vi "test Add State.vi"(8 "error in (no error)":errorcluster, 11 "TestCase in":refnum<class "Switch Scripting Unit Tests.lvclass">) -> (0 "error out":errorcluster, 3 "TestCase out":refnum<class "Switch Scripting Unit Tests.lvclass">)   [LabVIEW 2017, in "Switch Scripting.lvlib" / "Switch Scripting Unit Tests.lvclass"]
uses:
  Switch Scripting Unit Tests.lvclass
  Routing State.ctl
  Routing Channel/Connection.ctl
  Switch Scripting Unit Tests.lvclass/Switch Scripting Unit Tests.ctl
  <vilib>/addons/_JKI Toolkits/VI Tester/TestCase.llb/TestCase.lvclass
  Switch Scripting.lvlib
  C:/Program Files (x86)/National Instruments/LabVIEW 2017/vi.lib/addons/_JKI Toolkits/VI Tester/TestCase.llb/TestCase.lvclass
panel:
  in  "Save?":bool
  out "Output Filename":string
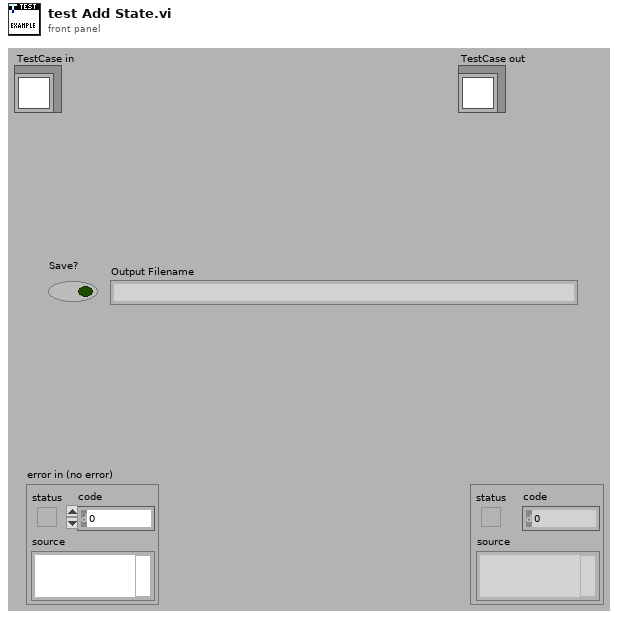
[diagram p1: front panel]
types:
  T1 = typedef "Switch Scripting.lvlib/Connection.ctl" = cluster{"source":string, "destination":string}
  T2 = typedef "Switch Scripting.lvlib/Routing State.ctl" = cluster{"name":string, "description":string, "value":i32, "connection list":T1[]}
  T3 = typedef "Custom Device API.lvlib/Custom Device Item Ref.ctl" = u64
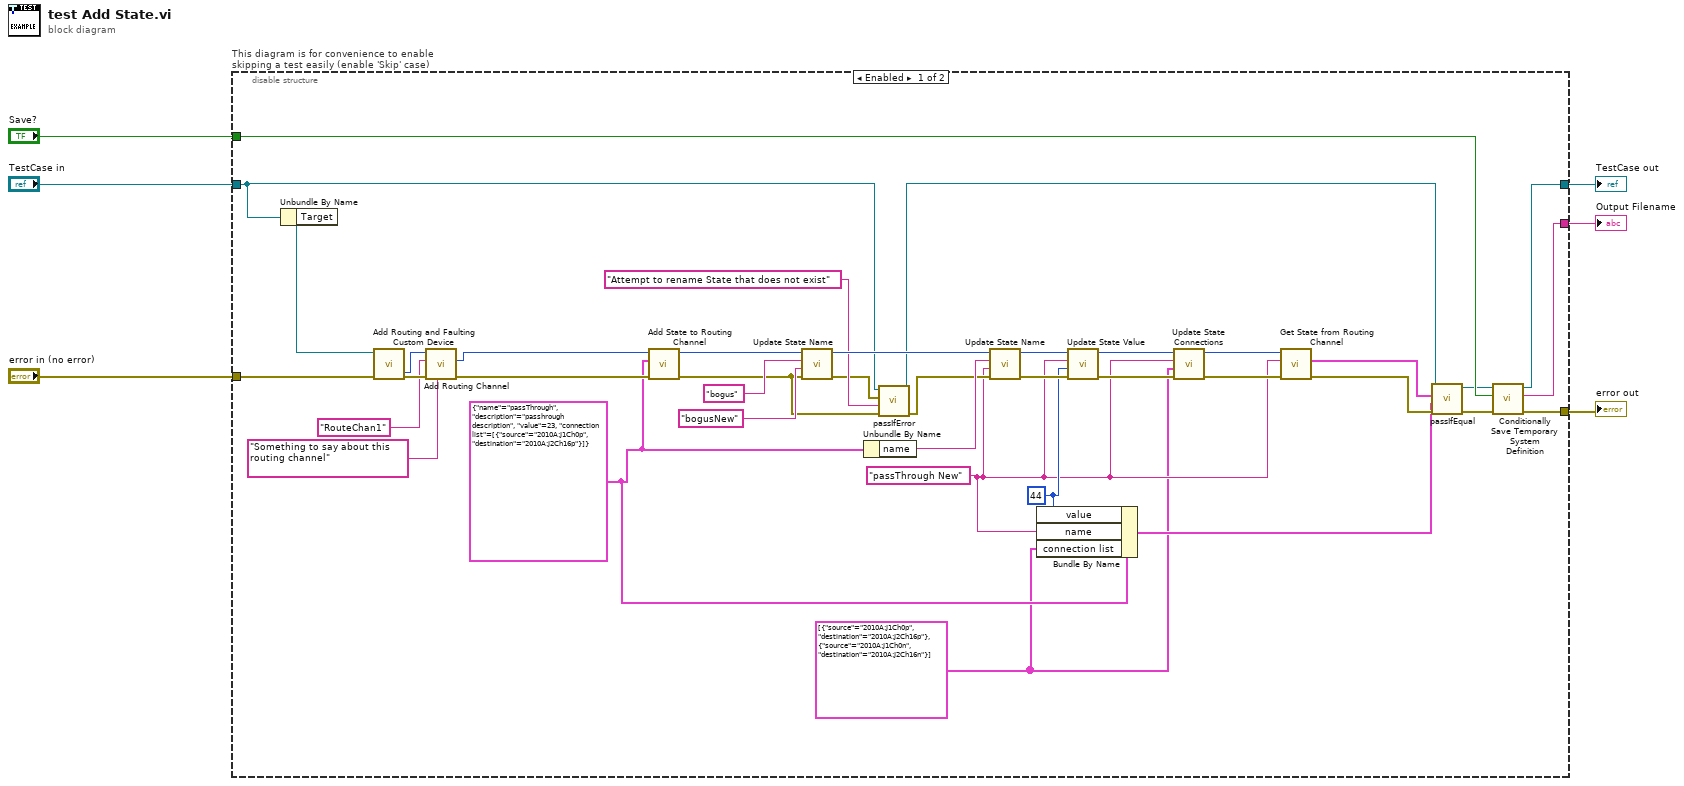
[diagram p0: block diagram]
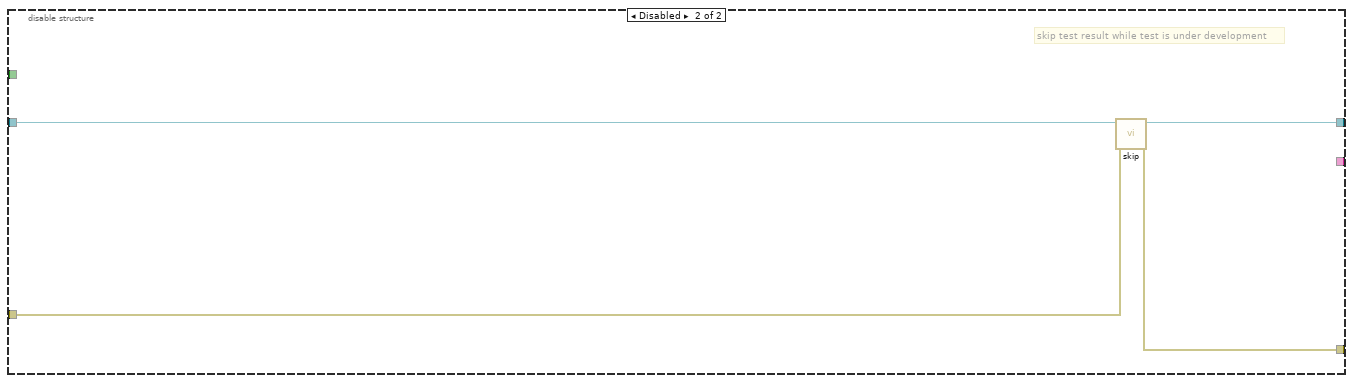
[diagram p2: hidden frame]
diagram:
  n1 = disable-structure "This diagram is for convenience to enable skipping a test easily (enable 'Skip' case)" shown="Enabled" {
    disable-tunnel: "TestCase in" -> [w16 w48]
    disable-tunnel: [w39 w46] -> w3
    disable-tunnel: [w43 w47] -> w5
    disable-tunnel: "error in (no error)" -> [w44 w45]
    disable-tunnel: [w42 _] -> w2
    disable-tunnel: "Save?" -> [w41 _]
    frame Enabled {
      w7 = T1[] [{"source"="2010A:J1Ch0p", "destination"="2010A:J2Ch16p"}, {"source"="2010A:J1Ch0n", "destination"="2010A:J2Ch16n"}] ("connection list")
      w26 = 44 ("New Value")
      w8 = "passThrough New" ("New State")
      w27 = T2 {"name"="passThrough", "description"="passhrough description", "value"=23, "connection list"=[{"source"="2010A:J1Ch0p", "destination"="2010A:J2Ch16p"}]} ("Routing State")
      n2 = Unbundle By Name(w16) -> ("Target"=w40:refnum<k24>)
      n3 = call "Add Routing and Faulting Custom Device.vi"("error in (no error)"=w44, "Target in"=w40) -> ("error out"=w38:errorcluster, "Routes Section Ref"=w35:T3)  [unwired: 5 in, 3 out]
      n4 = call "Add Routing Channel.vi"("Description"="Something to say about this routing channel", "error in (no error)"=w38, "Channel Name"="RouteChan1", "Routes Ref in"=w35) -> ("error out"=w32:errorcluster, "Channel Ref"=w31:T3)  [unwired: 5 in, 1 out]
      n5 = call "Add State to Routing Channel.vi"("error in (no error)"=w32, "Routing State"=w27, "Channel Ref in"=w31) -> ("error out"=w20:errorcluster, "Channel Ref out"=w24:T3)  [unwired: 7 in]
      n6 = call "Update State Name.vi"("error in (no error)"=w20, "New State"="bogusNew" ("State"), "State"="bogus", "Channel Ref in"=w24) -> ("error out"=w18:errorcluster, "Channel Ref out"=w23:T3)  [unwired: 6 in]
      n7 = Unbundle By Name(w27) -> ("name"=w30:string)
      n8 = call-dynamic "passIfError.vi"("error in (no error)"=w20, "task (\"\")"="Attempt to rename State that does not exist" ("custom report message (\"\")"), "error"=w18, "TestCase in"=w16) -> ("error out"=w17:errorcluster, "TestCase out"=w15:refnum<class "Switch Scripting Unit Tests.lvclass">)  [unwired: 6 in]
      n9 = call "Update State Name.vi"("error in (no error)"=w17, "New State"=w8, "State"=w30, "Channel Ref in"=w23) -> ("error out"=w28:errorcluster, "Channel Ref out"=w29:T3)  [unwired: 6 in]
      n10 = Bundle By Name(cluster=w27, "value"=w26, "name"=w8, "connection list"=w7) -> (w13:T2)
      n11 = call "Update State Value.vi"("error in (no error)"=w28, "New Value"=w26, "State"=w8, "Channel Ref in"=w29) -> ("error out"=w12:errorcluster, "Channel Ref out"=w10:T3)  [unwired: 6 in]
      n12 = call "Update State Connections.vi"("error in (no error)"=w12, "connection list"=w7, "State"=w8, "Channel Ref in"=w10) -> ("error out"=w11:errorcluster, "Channel Ref out"=w9:T3)  [unwired: 6 in]
      n13 = call "Get State from Routing Channel.vi"("error in (no error)"=w11, "State"=w8, "Channel Ref in"=w9) -> ("error out"=w25:errorcluster, "Routing State"=w14:T2)  [unwired: 6 in, 1 out]
      n14 = call-dynamic "passIfEqual.vi"("error in (no error)"=w25, "y"=w13, "x"=w14, "TestCase in"=w15) -> ("error out"=w37:errorcluster, "TestCase out"=w36:refnum<class "Switch Scripting Unit Tests.lvclass">)  [unwired: 6 in]
      n15 = call "Conditionally Save Temporary System Definition.vi"("error in (no error)"=w37, "Save?"=w41, "Test Case"=w36) -> ("error out"=w43:errorcluster, "filename"=w42:string, "Test Case"=w39:refnum<class "Switch Scripting Unit Tests.lvclass">)  [unwired: 6 in]
    }
    frame Disabled {
      # "skip test result while test is under development"
      n16 = call <vilib>:"skip.vi"("error in (no error)"=w45, "TestCase in"=w48) -> ("error out"=w47:errorcluster, "TestCase out"=w46:refnum<class "Switch Scripting Unit Tests.lvclass">)  [unwired: 8 in]
    }
  }
  "error out" <- w5
  "TestCase out" <- w3
  "Output Filename" <- w2
